vi "wait_for_notification.vi"(6 "ignore previous (T)":bool=TRUE, 8 "Error in":errorcluster caption="Error in (no error)", 9 "ms timeout (-1)":i32=-1, 10 "notifier":T1) -> (0 "Error out":errorcluster, 1 "timed out":bool, 2 "notifier duplicate":T1, 4 "notification":bool)   [LabVIEW 2015]
uses:
  cores/boolean_notifier.ctl
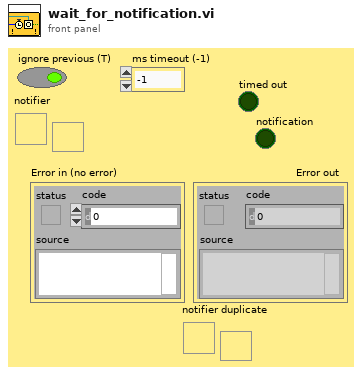
[diagram p1: front panel]
types:
  T1 = typedef "boolean_notifier.ctl" = refnum<notifier>
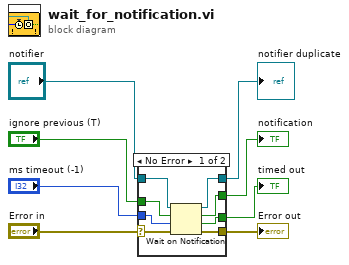
[diagram p0: block diagram]
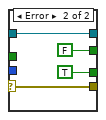
[diagram p2: hidden frame]
diagram:
  n1 = case shown="No Error" "Error in" {
    selector: "Error in" -> [w12 w20]
    tunnel: "ignore previous (T)" -> [w14 _]
    tunnel: "ms timeout (-1)" -> [w15 _]
    tunnel: [w13 TRUE] -> w6
    tunnel: [w11 w20] -> w4
    tunnel: "notifier" -> [w16 w18]
    tunnel: [w10 w18] -> w1
    tunnel: [w9 FALSE] -> w3
    frame No Error {
      n2 = Wait on Notification(notifier=w16, ignore previous (F)=w14, timeout in ms (-1)=w15, error in (no error)=w12) -> (notifier out=w10:T1, notification=w9:bool, timed out?=w13:bool, error out=w11:errorcluster)
    }
    frame Error {
    }
  }
  "timed out" <- w6
  "Error out" <- w4
  "notification" <- w3
  "notifier duplicate" <- w1
